vi "PH_gentec_Powermeter.set Wavelength.vi"(0 "i ref in":refnum<vi>, 2 "VISA resource in":refnum<visa-resource-name>, 4 "Device error in":errorcluster, 5 "error in":errorcluster) -> (13 "Settings changed?":bool, 14 "i ref out":refnum<vi>, 15 "Timeout":bool, 16 "VISA resource out":refnum<visa-resource-name>, 17 "Error Message":string, 18 "Device error out":errorcluster, 19 "error out":errorcluster)   [LabVIEW 2014, in "PH_gentec_Powermeter.lvlib"]
doc: "This VI sets the wavelength of the powermeter. Then the value verified by the powermeter is passed to own attributes and the GUI element."
uses:
  PH_gentec_Powermeter.lvlib
  non_GPL/instr.lib/gentec-SOLO-PE/gentec-SOLO-PE - Driver.lvlib
  PH_Powermeter_BaseClass/PH_Powermeter_BaseClass.lvlib
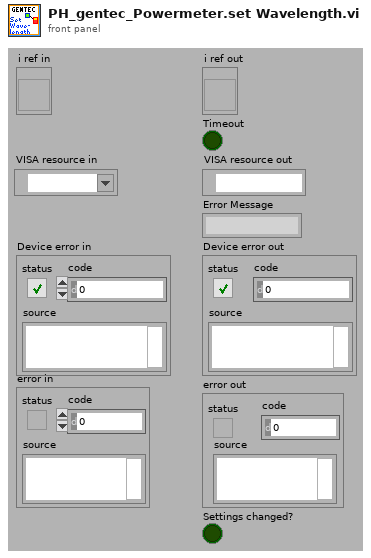
[diagram p1: front panel]
types:
  T1 = typedef "PH_Powermeter_BaseClass.lvlib/PH_Powermeter_BaseClass.i attribute.ctl" = cluster{"GUI References":T2, "Connection":T3, "Head Attributes":T5, "VISA resource":refnum<visa-resource-name>, "Energy":T6, "Service ID Energy":i32, "Wanted Settings":T7, "Current Settings":T7}
  T2 = typedef "PH_Powermeter_BaseClass.lvlib/PH_Powermeter_BaseClass.GUI Refs.ctl" = cluster{"Head Attributes":refnum<vi>, "Energy":refnum<vi>, "Connection":refnum<vi>, "VISA Resource":refnum<vi>, "Energy evolution":refnum<vi>, "Scaling Factor":refnum<vi>, "Range":refnum<vi>, "Wavelength":refnum<vi>, "Trigger Level":refnum<vi>, "Wanted Settings":refnum<vi>, "Current Settings":refnum<vi>}
  T3 = typedef "PH_Powermeter_BaseClass.lvlib/PH_Powermeter_BaseClass.Connection.ctl" = cluster{"failed checks":i8, "Timeout":bool, "Data read":string, "Failure":bool, "Error":bool, "State":T4}
  T4 = typedef "PH_Powermeter_BaseClass.lvlib/PH_Powermeter_BaseClass.State.ctl" = enum32{"off", "operating", "opened", "checked", "connected", "Sets to change", "running"}
  T5 = typedef "PH_Powermeter_BaseClass.lvlib/PH_Powermeter_BaseClass.Head Attributes.ctl" = cluster{"Instrument Type":string, "Head Version":string, "Head Name":string, "Serial Number":string, "Firmware":string, "Sensor Type":string, "MinimumRange":u32, "Maximum Range":u32, "Min Wavelength":i32, "Max Wavelength":i32}
  T6 = typedef "PH_Powermeter_BaseClass.lvlib/PH_Powermeter_BaseClass.Energy.ctl" = cluster{"current Value":dbl, "unscaled":dbl, "Scaling Factor":dbl}
  T7 = typedef "PH_Powermeter_BaseClass.lvlib/PH_gentec_BaseClass.Head Settings.ctl" = cluster{"Trigger Level":dbl, "Wavelength":u32, "Range":u32}
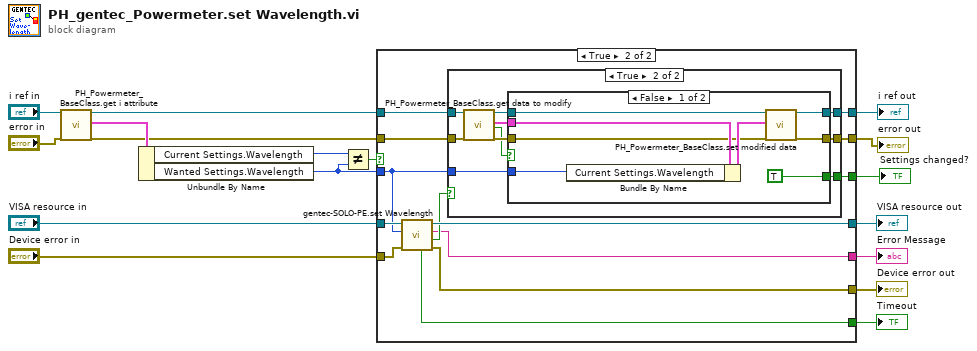
[diagram p0: block diagram]
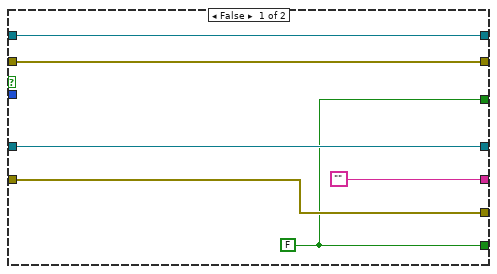
[diagram p2: hidden frame]
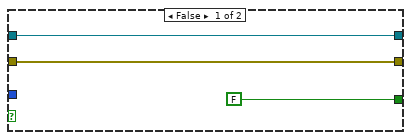
[diagram p3: hidden frame]
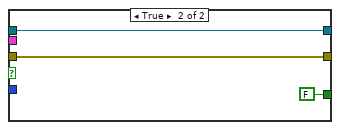
[diagram p4: hidden frame]
diagram:
  n1 = call "PH_Powermeter_BaseClass.get i attribute.vi"("i ref in"="i ref in", "error in (no error)"="error in") -> ("i ref out"=w9:refnum<vi>, "i attribute"=w13:T1, "error out"=w8:errorcluster)  [unwired: 15 in]
  n2 = Unbundle By Name(w13) -> ("Current Settings.Wavelength"=w12:u32, "Wanted Settings.Wavelength"=w11:u32)
  n3 = Not Equal?(x=w12, y=w11) -> (x != y?=w6:bool)
  n4 = case shown="True" w6 {
    tunnel: [w23 w36] -> w17
    tunnel: [w22 w35] -> w15
    tunnel: w11 -> [_ w29]
    tunnel: "VISA resource in" -> [w21 w33]
    tunnel: w9 -> [w23 w34]
    tunnel: w8 -> [w22 w30]
    tunnel: [w21 w28] -> w7
    tunnel: [w20 w31] -> w5
    tunnel: "Device error in" -> [w20 w32]
    tunnel: [w19 w27] -> w3
    tunnel: ["" w25] -> w1
    tunnel: [w19 w24] -> w2
    frame False {
      w19 = FALSE ("Timeout")
    }
    frame True {
      n5 = call "gentec-SOLO-PE.set Wavelength.vi"("error in (no error)"=w32, "Wavelength [nm]"=w29, "VISA Refnum in"=w33) -> ("error out"=w31:errorcluster, "Acknoledged?"=w26:bool, "Error"=w25:string, "VISA Refnum out"=w28:refnum<visa-resource-name>, "Timeout"=w24:bool)  [unwired: 4 in]
      n6 = case shown="True" w26 {
        tunnel: [w39 w45] -> w36
        tunnel: [w38 w44] -> w35
        tunnel: w34 -> [w39 w43]
        tunnel: w30 -> [w38 w42]
        tunnel: w29 -> [_ w41]
        tunnel: [FALSE w40] -> w27
        frame False {
        }
        frame True {
          n7 = call "PH_Powermeter_BaseClass.get data to modify.vi"("i ref in"=w43, "error in (no error)"=w42) -> ("i ref out"=w49:refnum<vi>, "i attribute"=w48:T1, "timed out"=w46:bool, "error out"=w47:errorcluster)  [unwired: 14 in]
          n8 = case shown="False" w46 {
            tunnel: w47 -> [w54 w59]
            tunnel: w49 -> [w57 w60]
            tunnel: [w52 w60] -> w45
            tunnel: [w51 w59] -> w44
            tunnel: w48 -> [w56 _]
            tunnel: w41 -> [w50 _]
            tunnel: [TRUE FALSE] -> w40
            frame False {
              n9 = Bundle By Name(cluster=w56, "Current Settings.Wavelength"=w50) -> (w55:T1)
              n10 = call "PH_Powermeter_BaseClass.set modified data.vi"("i ref in"=w57, "i attribute"=w55, "error in (no error)"=w54) -> ("i ref out"=w52:refnum<vi>, "error out"=w51:errorcluster)  [unwired: 15 in]
            }
            frame True {
            }
          }
        }
      }
    }
  }
  "error out" <- w15
  "i ref out" <- w17
  "VISA resource out" <- w7
  "Device error out" <- w5
  "Settings changed?" <- w3
  "Timeout" <- w2
  "Error Message" <- w1
